vi "init.vi"(8 "error in (no error)":errorcluster, 10 "sdf path":string, 11 "abstract-tree in":refnum<class "abstract-tree.lvclass">) -> (0 "error out":errorcluster, 3 "abstract-tree out":refnum<class "abstract-tree.lvclass">)   [LabVIEW 2017, in "vs-tree-utility.lvlib" / "abstract-tree.lvclass"]
uses:
  abstract-tree.lvclass
  NationalInstruments.VeriStand.SystemDefinitionAPI
  abstract-tree.lvclass/abstract-tree.ctl
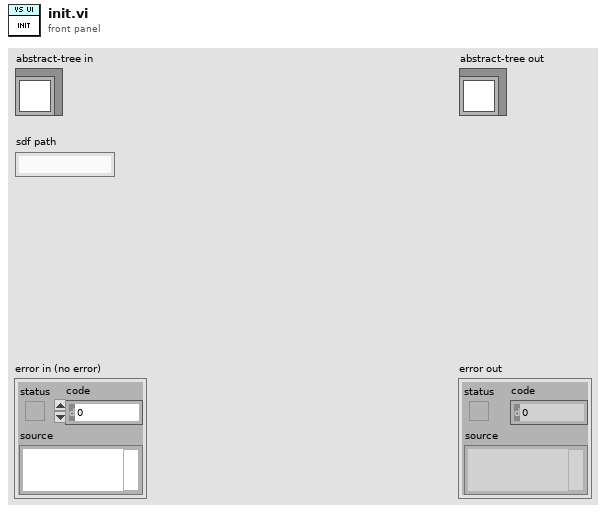
[diagram p1: front panel]
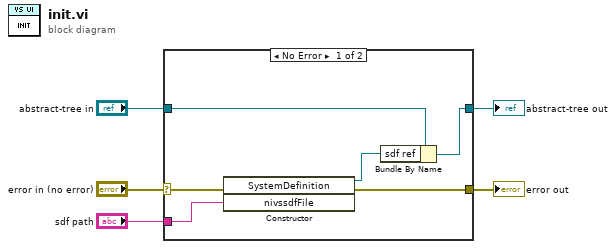
[diagram p0: block diagram]
diagram:
  n1 = case shown="No Error" "error in (no error)" {
    selector: "error in (no error)" -> [w11 w13]
    tunnel: [w9 w13] -> w4
    tunnel: [w6 w12] -> w2
    tunnel: "abstract-tree in" -> [w10 w12]
    tunnel: "sdf path" -> [w8 _]
    frame No Error {
      n2 = constructor class="SystemDefinition"(error in=w11, "nivssdfFile"=w8) -> (reference out=w7:refnum<k24>, error out=w9:errorcluster)  [unwired: 2 in, 2 out]
      n3 = Bundle By Name(cluster=w10, "sdf ref"=w7) -> (w6:refnum<class "abstract-tree.lvclass">)
    }
    frame Error {
    }
  }
  "error out" <- w4
  "abstract-tree out" <- w2
